vi "pcap-write.vi"(1 "Data to Write":string) -> (0 "Write Error":bool)   [LabVIEW 2017]
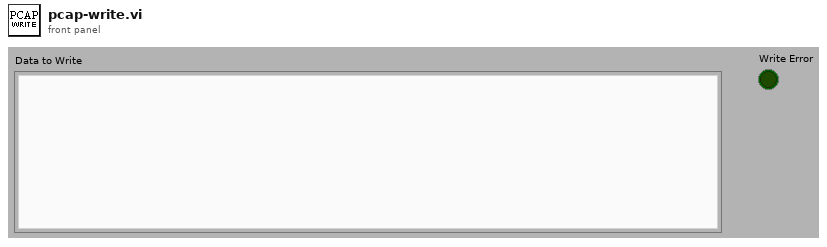
[diagram p1: front panel]
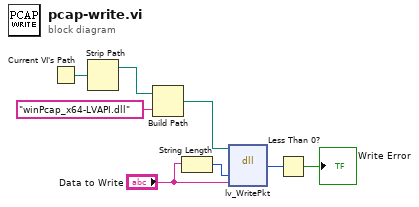
[diagram p0: block diagram]
diagram:
  n1 = Current VI's Path() -> (path=w4:path)
  n2 = Strip Path(path=w4) -> (stripped path=w3:path)  [unwired: 1 out]
  n3 = Build Path(base path=w3, name or relative path="winPcap_x64-LVAPI.dll") -> (appended path=w1:path)
  n4 = String Length(string="Data to Write") -> (length=w8:i32)
  n5 = dll-call lib="C:/Users/ucbtspu.AD/OneDrive - University College London/Local SCC/SilverLab-Microscope x64/Ethernet/winPcap_x64-LVAPI.dll" fn="lv_WritePkt"(path in=w1, w8, "Data to Write") -> ("return type"=w7:i32)  [unwired: 4 in, 2 out]
  n6 = Less Than 0?(x=w7) -> (x < 0?=→"Write Error":bool)
